vi "Get Chars Array.vi"(7 "Width":i32, 8 "error in (no error)":errorcluster, 11 "Lines":refnum<class "TermLine.lvclass">[](array[class])) -> (0 "error out":errorcluster, 2 "TermChars":T1[][](array[typedef]))   [LabVIEW 2020, in "Terminal.lvlib" / "TermLine.lvclass"]
uses:
  TermLine.lvclass
  TermLine.lvclass/TermLine.ctl
  Term Char.ctl
  Terminal.lvlib
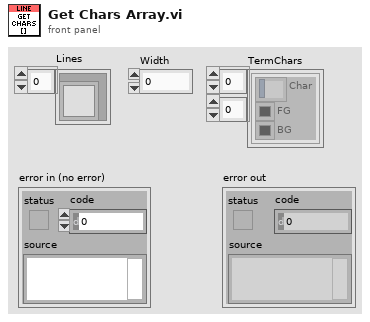
[diagram p1: front panel]
types:
  T1 = typedef "Terminal.lvlib/Term Char.ctl" = cluster{"Char":string, "FG":u32, "BG":u32}
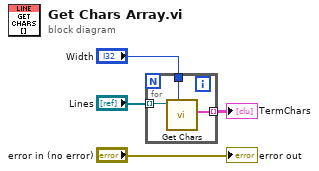
[diagram p0: block diagram]
diagram:
  n1 = for {
    tunnel: "Lines" -> [w7] mode=indexing
    tunnel: "Width" -> [w6]
    tunnel: [w5] -> w1 mode=indexing
    n2 = call "Get Chars.vi"("Width"=w6, "TermLine in"=w7) -> ("TermChars"=w5:T1[])  [unwired: 7 in, 2 out]
  }
  "TermChars" <- w1
  "error out" <- "error in (no error)"
